vi "MulticolorBoxPruebas.vi"() -> ()   [LabVIEW 2020]
panel:
  in  "stop":bool
  in  "Multicolumn Listbox":i32(listbox)
  out "subarray":string[](array[string])
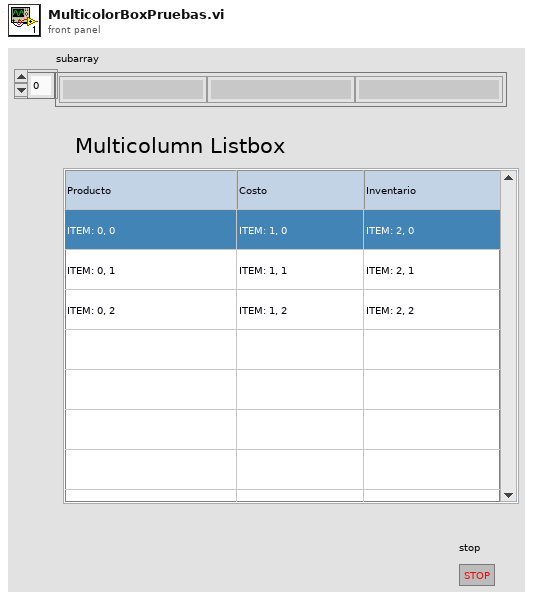
[diagram p1: front panel]
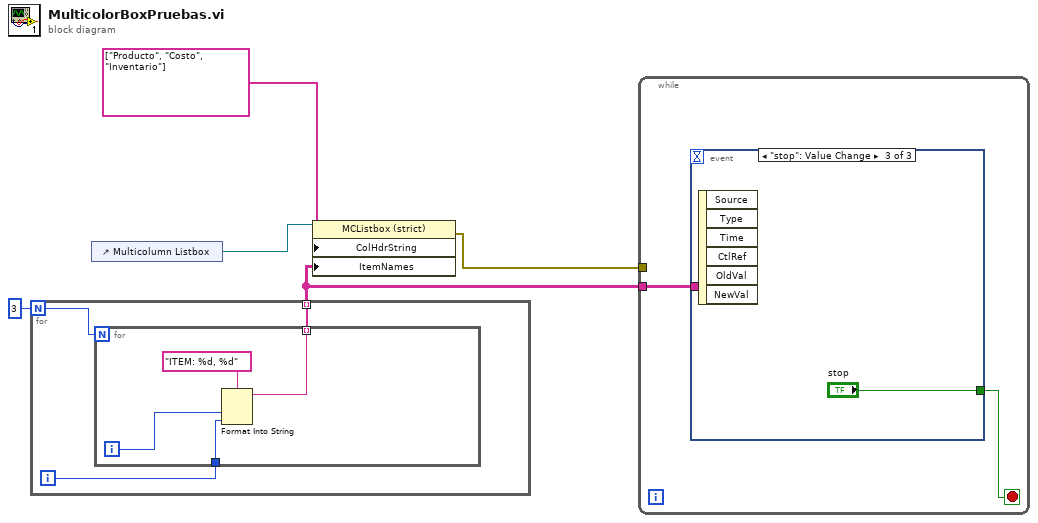
[diagram p0: block diagram]
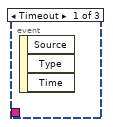
[diagram p2: hidden frame]
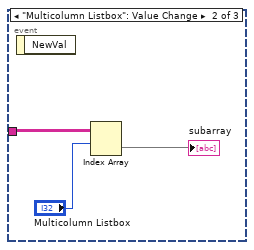
[diagram p3: hidden frame]
diagram:
  n1 = for {
    N: 3 -> [w8]
    tunnel: [w7] -> w1 mode=indexing
    i -> [w6]
    n2 = for {
      N: w8 -> [_]
      tunnel: [w11] -> w7 mode=indexing
      tunnel: w6 -> [w9]
      i -> [w12]
      n3 = Format Into String(format string="ITEM: %d, %d", w12, w9) -> (resulting string=w11:string)  [unwired: 2 in, 1 out]
    }
  }
  n4 = control-ref of="Multicolumn Listbox"() -> (w5:refnum<vi>)
  n5 = property class="MCListbox (strict)"(reference=w5, "ColHdrString"=string[] ["Producto", "Costo", "Inventario"] ("Column Header Strings[]"), "ItemNames"=w1) -> (error out=w2:errorcluster)  [unwired: 1 in, 1 out]
  n6 = while {
    tunnel: w2 -> [_]
    tunnel: w1 -> [w14]
    stop <- w13 stop-if-true
    n7 = event shown="[2] \"stop\": Value Change" {
      selector: _ -> [_ _ _]
      dyn-events: _ -> [_ _ _]
      timeout: _ -> [_ _ _]
      tunnel: w14 -> [_ w17 _]
      tunnel: [_ _ "stop"] -> w13
      event Timeout {
        n8 = event-data() -> ()  [unwired: 1 in, 3 out]
      }
      event "Multicolumn Listbox": Value Change {
        n9 = event-data() -> ()  [unwired: 1 in, 1 out]
        n10 = Index Array(array=w17, index (row)="Multicolumn Listbox") -> (element=→"subarray":string[])  [unwired: 1 in]
      }
      event "stop": Value Change {
        n11 = event-data() -> ()  [unwired: 1 in, 6 out]
      }
    }
  }
